vi "subHamamatsu_ApplyDAQwaveform.vi"(5 "Camera info":cluster{"Handle in":u32, "Image file path":path}, 6 "Acquisition params":T1={"Sampling rate (Hz)"=0.0, "dt (sec)"=0.0, "total time (sec)"=0.0, "# samples"=0, "Exposure time (ms)"=1000.0, "# frames"=0} {"Exposure time (ms)" format="%0.5f"; "Sampling rate (Hz)" format="%#.3f"}, 7 "Waveform port selection":T2={"Dev2 DO lines"=["Dev2/port0/line3", "Dev2/port0/line5"], "Dev2 AO lines"=["Dev2/ao3", "Dev2/ao5"], "Patch AO line"="Dev1/ao0", "Dev1 AI lines"=["Dev1/ai0", "Dev1/ai8"], "Dev1 timing DO"="Dev1/port0/line1", "Camera timing DI"="Dev1/port0/line0", "Dev1 trigger source"="/Dev1/PFI0", "Dev2 trigger source"="/Dev2/PFI0"}, 8 "Camera in (no error)":errorcluster, 9 "Dev1 AO waveform":waveform(dbl)(graph)={"t0"=timestamp(0 s since 1904-01-01), "dt"=0.1, "Y"=array[20000 elements]}, 10 "Dev2 AO waveform":waveform(dbl)[](graph)=[{"t0"=timestamp(0 s since 1904-01-01), "dt"=0.1, "Y"=array[20000 elements]}, {"t0"=timestamp(0 s since 1904-01-01), "dt"=0.1, "Y"=array[20000 elements]}], 11 "Dev2 DO waveform":digitalwaveform[](graph)=[{"t0"=timestamp(0 s since 1904-01-01), "dt"=0.1, "Y"={"transitions"=[0, 10000, 19999], "data"=[[1], [0], [0]]}}, {"t0"=timestamp(0 s since 1904-01-01), "dt"=0.1, "Y"={"transitions"=[0, 10000, 19999], "data"=[[0], [1], [1]]}}]) -> (0 "Camera out":errorcluster, 2 "AI Waveform":dbl[][](graph), 3 "Camera timging DI":digitalwaveform(graph))   [LabVIEW 2015]
uses:
  <vilib>/DAQmx/write.llb/DAQmx Write (Analog Wfm 1Chan NSamp).vi
  <vilib>/DAQmx/write.llb/DAQmx Write (Analog 1D Wfm NChan NSamp).vi
  <vilib>/DAQmx/write.llb/DAQmx Write (Digital 1D Wfm NChan NSamp).vi
  <vilib>/DAQmx/write.llb/DAQmx Write (Digital Wfm 1Chan NSamp).vi
  <vilib>/DAQmx/read.llb/DAQmx Read (Analog 2D DBL NChan NSamp).vi
  <vilib>/DAQmx/read.llb/DAQmx Read (Digital Wfm 1Chan NSamp).vi
  <vilib>/DAQmx/create/channels.llb/DAQmx Create Channel (DO-Digital Output).vi
  <vilib>/Waveform/DWDTOps.llb/DWDT Analog to Digital.vi
  <vilib>/DAQmx/create/channels.llb/DAQmx Create Channel (DI-Digital Input).vi
  <vilib>/DAQmx/create/channels.llb/DAQmx Create Channel (AO-Voltage-Basic).vi
  <vilib>/DAQmx/create/channels.llb/DAQmx Create Channel (AI-Voltage-Basic).vi
  <vilib>/DAQmx/configure/timing.llb/DAQmx Timing (Sample Clock).vi
  <vilib>/DAQmx/miscellaneous.llb/DAQmx Fill In Error Info.vi
  <vilib>/DAQmx/configure/trigger.llb/DAQmx Start Trigger (Digital Edge).vi
  <vilib>/Waveform/DWDTOps.llb/DWDT Uncompress Digital.vi
  <resource>/objmgr/daqmx.rc
panel:
  out "Dev1 SampClk.Rate":dbl format="%#.3f"
  out "Dev2 SampClk.Rate":dbl format="%#.3f"
  out "Dev1 timing DO":digitalwaveform(graph)={"t0"=timestamp(0 s since 1904-01-01), "dt"=0.1, "Y"={"transitions"=[0, 19999], "data"=[[1], [1]]}}
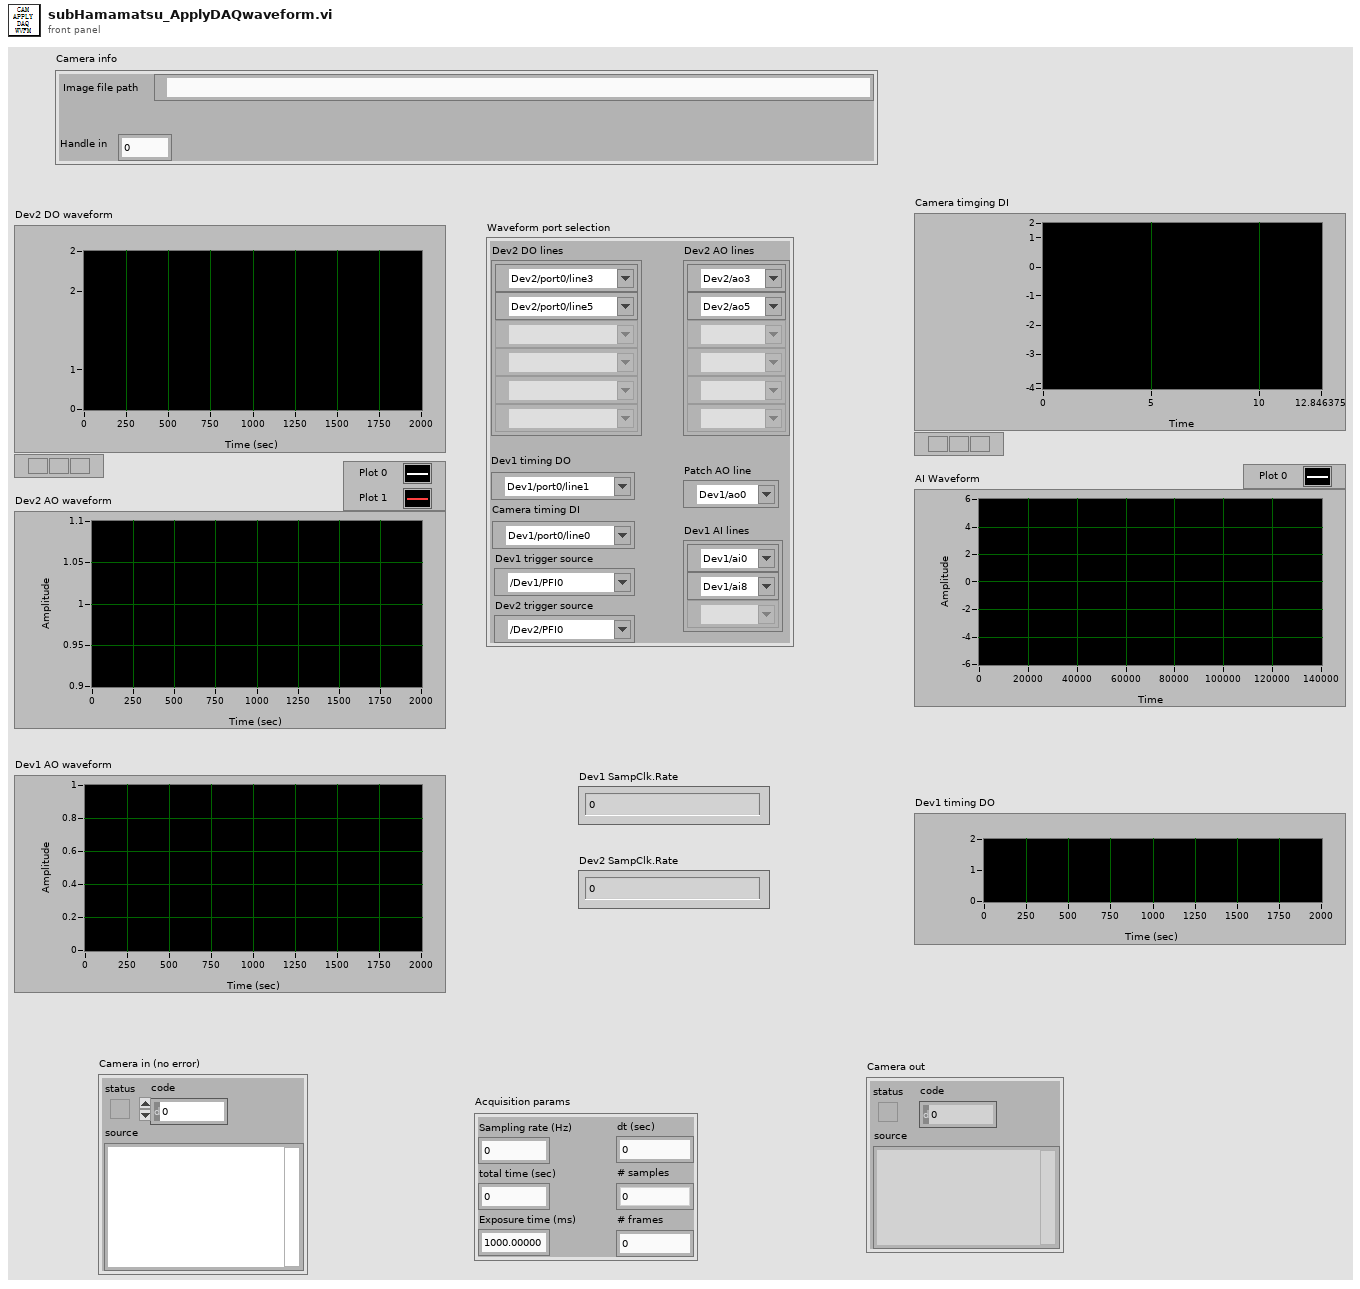
[diagram p1: front panel]
types:
  T1 = cluster{"Sampling rate (Hz)":dbl, "dt (sec)":dbl, "total time (sec)":dbl, "# samples":i32, "Exposure time (ms)":dbl, "# frames":i32}
  T2 = cluster{"Dev2 DO lines":tag[], "Dev2 AO lines":tag[], "Patch AO line":tag, "Dev1 AI lines":tag[], "Dev1 timing DO":tag, "Camera timing DI":tag, "Dev1 trigger source":tag, "Dev2 trigger source":tag}
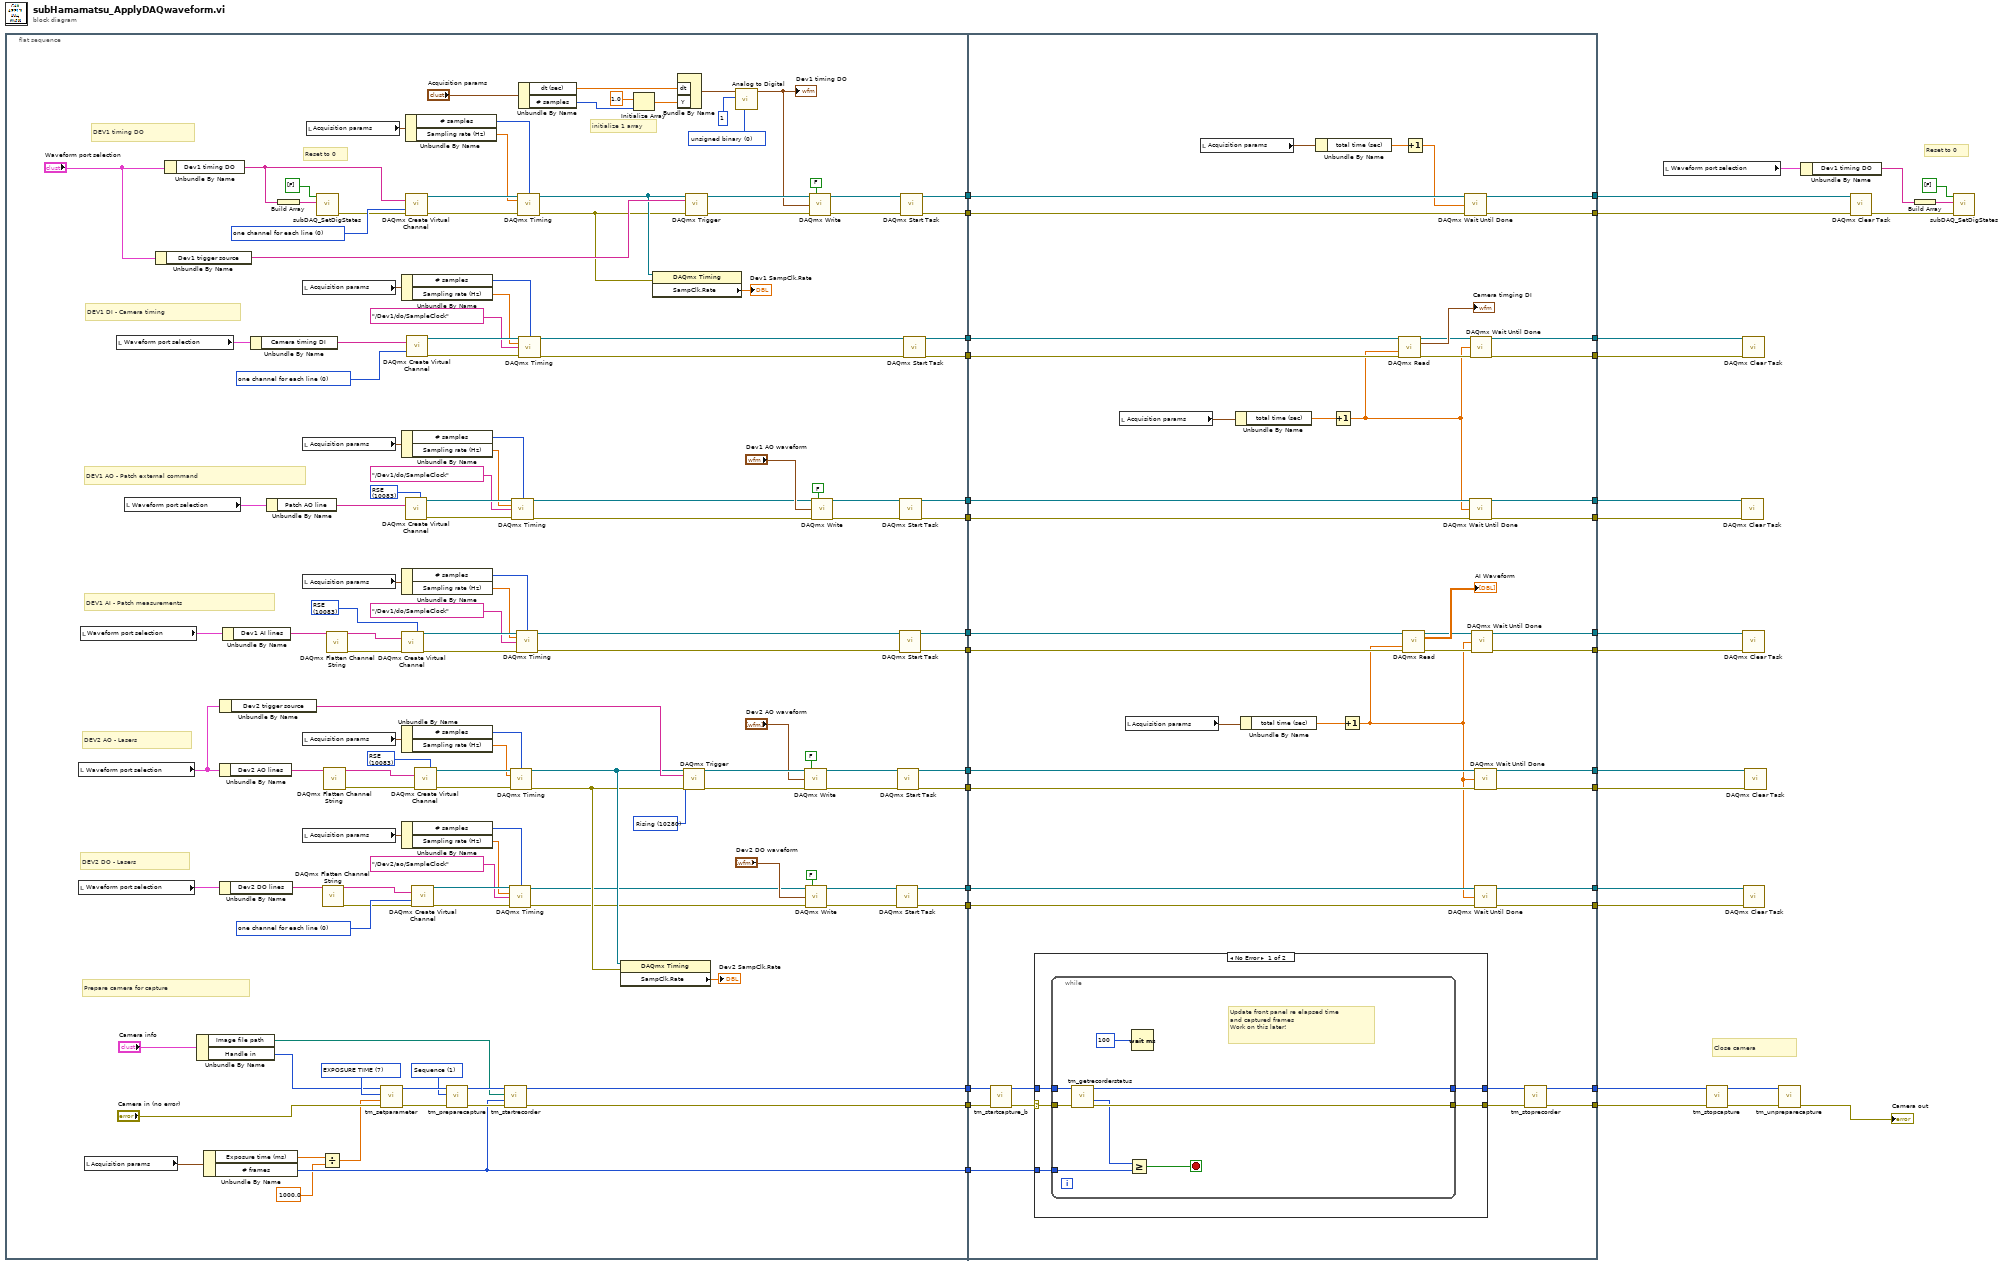
[diagram p0: block diagram]
diagram:
  # "Close camera"
  # "Reset to 0"
  n1 = flat-sequence {
    tunnel: [w155] -> w29
    tunnel: [w142] -> w28
    tunnel: [w141] -> w27
    tunnel: [w133] -> w26
    tunnel: [w122] -> w25
    tunnel: [w121] -> w24
    tunnel: [w114] -> w23
    tunnel: [w113] -> w22
    tunnel: [w110] -> w21
    tunnel: [w109] -> w20
    tunnel: [w106] -> w19
    tunnel: [w105] -> w18
    tunnel: [w91] -> w17
    tunnel: [w90] -> w16
    tunnel: [w65] -> w1
    tunnel: w29 -> [w204]
    tunnel: w28 -> [w206]
    tunnel: w27 -> [w205]
    tunnel: w26 -> [w203]
    tunnel: w25 -> [w202]
    tunnel: w24 -> [w201]
    tunnel: w23 -> [w199]
    tunnel: w22 -> [w200]
    tunnel: w21 -> [w198]
    tunnel: w20 -> [w197]
    tunnel: w19 -> [w196]
    tunnel: w18 -> [w195]
    tunnel: w17 -> [w216]
    tunnel: w16 -> [w215]
    tunnel: [w214] -> w15
    tunnel: [w213] -> w14
    tunnel: [w194] -> w13
    tunnel: [w193] -> w12
    tunnel: [w192] -> w11
    tunnel: [w191] -> w10
    tunnel: [w190] -> w9
    tunnel: [w189] -> w8
    tunnel: [w188] -> w7
    tunnel: [w187] -> w6
    tunnel: [w186] -> w5
    tunnel: [w185] -> w4
    tunnel: [w184] -> w3
    tunnel: [w183] -> w2
    tunnel: w1 -> [w182]
    frame #0 {
      w58 = 10083 items=["Default"=-1, "RSE"=10083, "Differential"=10106, "Pseudodifferential"=12529] ("output terminal configuration")
      w59 = 10083 items=["Default"=-1, "RSE"=10083, "Differential"=10106, "Pseudodifferential"=12529] ("output terminal configuration")
      w60 = 10083 items=["Default"=-1, "RSE"=10083, "NRSE"=10078, "Differential"=10106, "Pseudodifferential"=12529] ("input terminal configuration")
      w63 = 10280 items=["Rising"=10280, "Falling"=10171] ("edge")
      w89 = u16 0 items=["unsigned binary", "offset binary", "2's complement"] ("data format (offset binary)")
      w95 = 7 items=["BINNING"=1, "BITS PER CHANNEL"=2, "ACTIVE VIEW INDEX"=3, "CCD MODE"=4, "SENSOR MODE"=5, "READOUT MODE"=6, "EXPOSURE TIME"=7, "CONTRAST GAIN"=8, "CONTRAST OFFSET"=9, "LIGHT MODE"=10, "SENSITIVITY"=11, "WHITE BALANCE"=12, "PHOTON IMAGING MODE"=13, "HIGH DYNAMIC RANGE MODE"=14, "TRIGGER SOURCE"=15, "TRIGGER ACTIVE"=16, "TRIGGER MODE"=17, "TRIGGER POLARITY"=18, "TRIGGER GLOBAL EXPOSURE"=19, "FIRST TRIGGER BEHAVIOR"=20, "TRIGGER TIMES"=21, "OUTPUT TRIGGER POLARITY"=22, "OUTPUT TRIGGER DELAY"=23, "OUTPUT TRIGGER PERIOD"=24, "TEMPERATURE"=25, "TEMPERATURE TARGET"=26, "SENSOR COOLER FAN"=27, "MECHANICAL SHUTTER"=28, "BACK FOCUS POSITION"=29, "FRAMEBUNDLE MODE"=30, "FRAMEBUNDLE NUMBER"=31, "LINEBUNDLE HEIGHT"=32, "TRIGGER CONNECTOR"=33, "IMAGE PIXEL TYPE"=34] ("Parameter")
      w92 = 1 items=["Snap", "Sequence"] ("Capture mode")
      w146 = 0 items=["one channel for each line", "one channel for all lines"] ("line grouping")
      w159 = 0 items=["one channel for each line", "one channel for all lines"] ("line grouping")
      w172 = 0 items=["one channel for each line", "one channel for all lines"] ("line grouping")
      # "Prepare camera for capture"
      # "Reset to 0"
      # "DEV2 DO - Lasers"
      # "DEV2 AO - Lasers"
      # "DEV1 AI - Patch measurements"
      # "DEV1 AO - Patch external command"
      # "DEV1 DI - Camera timing"
      # "DEV1 timing DO"
      # "initialize 1 array"
      n2 = local read "Waveform port selection"() -> (w86:T2)
      n3 = local read "Waveform port selection"() -> (w108:T2)
      n4 = local read "Waveform port selection"() -> (w116:T2)
      n5 = local read "Acquisition params"() -> (w66:T1)
      n6 = local read "Waveform port selection"() -> (w135:T2)
      n7 = local read "Waveform port selection"() -> (w127:T2)
      n8 = Unbundle By Name("Waveform port selection") -> ("Dev1 trigger source"=w83:tag)
      n9 = Unbundle By Name("Waveform port selection") -> ("Dev1 timing DO"=w103:tag)
      n10 = Unbundle By Name("Camera info") -> ("Image file path"=w87:path, "Handle in"=w64:u32)
      n11 = Unbundle By Name(w66) -> ("Exposure time (ms)"=w39:dbl, "# frames"=w65:i32)
      n12 = Unbundle By Name(w86) -> ("Dev2 AO lines"=w111:tag[])
      n13 = Unbundle By Name(w108) -> ("Dev2 DO lines"=w107:tag[])
      n14 = Unbundle By Name(w86) -> ("Dev2 trigger source"=w85:tag)
      n15 = Unbundle By Name(w116) -> ("Dev1 AI lines"=w115:tag[])
      n16 = Unbundle By Name(w135) -> ("Camera timing DI"=w134:tag)
      n17 = Unbundle By Name(w127) -> ("Patch AO line"=w125:tag)
      n18 = Build Array(w103) -> (w102:tag[])
      n19 = local read "Acquisition params"() -> (w81:T1)
      n20 = local read "Acquisition params"() -> (w76:T1)
      n21 = local read "Acquisition params"() -> (w75:T1)
      n22 = local read "Acquisition params"() -> (w74:T1)
      n23 = local read "Acquisition params"() -> (w73:T1)
      n24 = local read "Acquisition params"() -> (w43:T1)
      n25 = call "subDAQ_SetDigStates.vi"("Digital line array"=w102, "Digital States (Value) array"=bool[] [FALSE] ("Digital state array")) -> ("Error out"=w104:errorcluster)  [unwired: 9 in]
      n26 = Divide(x=w39, y=1000.0) -> (x/y=w40:dbl)
      n27 = call <vilib>:"DAQmx Flatten Channel String.vi"("names in"=w107) -> ("names out"=w170:string, "error out"=w169:errorcluster)  [unwired: 13 in]
      n28 = call <vilib>:"DAQmx Flatten Channel String.vi"("names in"=w111) -> ("names out"=w151:string, "error out"=w152:errorcluster)  [unwired: 13 in]
      n29 = call <vilib>:"DAQmx Flatten Channel String.vi"("names in"=w115) -> ("names out"=w120:string, "error out"=w119:errorcluster)  [unwired: 13 in]
      n30 = call "tm_setparameter.vi"("error in (no error)"="Camera in (no error)", "Value in"=w40, "Parameter"=w95, "Handle in"=w64) -> ("error out"=w97:errorcluster, "Handle out"=w96:u32)  [unwired: 6 in]
      n31 = Unbundle By Name(w81) -> ("# samples"=w80:i32, "Sampling rate (Hz)"=w79:dbl)
      n32 = Unbundle By Name(w76) -> ("# samples"=w78:i32, "Sampling rate (Hz)"=w77:dbl)
      n33 = Unbundle By Name(w75) -> ("# samples"=w67:i32, "Sampling rate (Hz)"=w68:dbl)
      n34 = call-poly <vilib>:"DAQmx Create Virtual Channel.vi"("input terminal configuration"=w60, "physical channels"=w120, "error in"=w119) -> ("task out"=w117:refnum<k21>, "error out"=w118:errorcluster)  [unwired: 11 in]
      n35 = Unbundle By Name(w74) -> ("# samples"=w69:i32, "Sampling rate (Hz)"=w70:dbl)
      n36 = Unbundle By Name(w73) -> ("# samples"=w72:i32, "Sampling rate (Hz)"=w71:dbl)
      n37 = Unbundle By Name(w43) -> ("# samples"=w42:i32, "Sampling rate (Hz)"=w41:dbl)
      n38 = call-poly <vilib>:"DAQmx Create Virtual Channel.vi"("output terminal configuration"=w59, "physical channels"=w125) -> ("task out"=w128:refnum<k21>, "error out"=w130:errorcluster)  [unwired: 12 in]
      n39 = call-poly <vilib>:"DAQmx Create Virtual Channel.vi"("lines"=w103, "line grouping"=w146, "error in"=w104) -> ("task out"=w147:refnum<k21>, "error out"=w150:errorcluster)  [unwired: 11 in]
      n40 = call-poly <vilib>:"DAQmx Create Virtual Channel.vi"("lines"=w134, "line grouping"=w159) -> ("task out"=w158:refnum<k21>, "error out"=w157:errorcluster)  [unwired: 12 in]
      n41 = call-poly <vilib>:"DAQmx Create Virtual Channel.vi"("lines"=w170, "line grouping"=w172, "error in"=w169) -> ("task out"=w171:refnum<k21>, "error out"=w166:errorcluster)  [unwired: 11 in]
      n42 = call-poly <vilib>:"DAQmx Create Virtual Channel.vi"("output terminal configuration"=w58, "physical channels"=w151, "error in"=w152) -> ("task out"=w165:refnum<k21>, "error out"=w161:errorcluster)  [unwired: 11 in]
      n43 = call "tm_preparecapture.vi"("error in (no error)"=w97, "Capture mode"=w92, "Handle in"=w96) -> ("error out"=w93:errorcluster, "Handle out"=w94:u32)  [unwired: 5 in, 2 out]
      n44 = call "tm_startrecorder.vi"("error in (no error)"=w93, "frames"=w65, "File"=w87, "Handle in"=w94) -> ("error out"=w90:errorcluster, "Handle out"=w91:u32)  [unwired: 6 in]
      n45 = call-poly <vilib>:"DAQmx Timing.vi"("task/channels in"=w171, "samples per channel"=w72, "rate"=w71, "source"=tag "/Dev2/ao/SampleClock", "error in"=w166) -> ("task out"=w45:refnum<k21>, "error out"=w44:errorcluster)  [unwired: 9 in]
      n46 = call-poly <vilib>:"DAQmx Timing.vi"("task/channels in"=w165, "samples per channel"=w69, "rate"=w70, "error in"=w161) -> ("task out"=w52:refnum<k21>, "error out"=w51:errorcluster)  [unwired: 10 in]
      n47 = call-poly <vilib>:"DAQmx Timing.vi"("task/channels in"=w128, "samples per channel"=w78, "rate"=w77, "source"=tag "/Dev1/do/SampleClock", "error in"=w130) -> ("task out"=w55:refnum<k21>, "error out"=w54:errorcluster)  [unwired: 9 in]
      n48 = call-poly <vilib>:"DAQmx Timing.vi"("task/channels in"=w117, "samples per channel"=w67, "rate"=w68, "source"=tag "/Dev1/do/SampleClock", "error in"=w118) -> ("task out"=w47:refnum<k21>, "error out"=w46:errorcluster)  [unwired: 9 in]
      n49 = call-poly <vilib>:"DAQmx Timing.vi"("task/channels in"=w147, "samples per channel"=w42, "rate"=w41, "error in"=w150) -> ("task out"=w49:refnum<k21>, "error out"=w48:errorcluster)  [unwired: 10 in]
      n50 = Unbundle By Name("Acquisition params") -> ("dt (sec)"=w61:dbl, "# samples"=w62:i32)
      n51 = call-poly <vilib>:"DAQmx Timing.vi"("task/channels in"=w158, "samples per channel"=w80, "rate"=w79, "source"=tag "/Dev1/do/SampleClock", "error in"=w157) -> ("task out"=w57:refnum<k21>, "error out"=w56:errorcluster)  [unwired: 9 in]
      n52 = property class="DAQmx Timing"(reference=w52, error in=w51) -> ("SampClk.Rate"=→"Dev2 SampClk.Rate":dbl)  [unwired: 2 out]
      n53 = Initialize Array(1.0 ("element"), w62) -> (w139:dbl[])
      n54 = property class="DAQmx Timing"(reference=w49, error in=w48) -> ("SampClk.Rate"=→"Dev1 SampClk.Rate":dbl)  [unwired: 2 out]
      n55 = Bundle By Name("dt"=w61, "Y"=w139) -> (w137:waveform(dbl))  [unwired: 1 in]
      n56 = call-poly <vilib>:"DAQmx Trigger.vi"("task/channels in"=w52, "source"=w85, "edge"=w63, "error in"=w51) -> ("task out"=w163:refnum<k21>, "error out"=w162:errorcluster)  [unwired: 10 in]
      n57 = call-poly <vilib>:"DAQmx Trigger.vi"("task/channels in"=w49, "source"=w83, "error in"=w48) -> ("task out"=w144:refnum<k21>, "error out"=w145:errorcluster)  [unwired: 11 in]
      n58 = call-poly <vilib>:"Analog to Digital.vi"("data format (offset binary)"=w89, "resolution (16 bit)"=1, "analog waveform"=w137) -> ("digital waveform"=w136:digitalwaveform)  [unwired: 5 in, 3 out]
      "Dev1 timing DO" <- w136
      n59 = call-poly <vilib>:"DAQmx Write.vi"("task/channels in"=w163, "auto start"=FALSE, "data"="Dev2 AO waveform", "error in"=w162) -> ("task out"=w164:refnum<k21>, "error out"=w112:errorcluster)  [unwired: 9 in, 1 out]
      n60 = call-poly <vilib>:"DAQmx Write.vi"("task/channels in"=w45, "auto start"=FALSE, "data"="Dev2 DO waveform", "error in"=w44) -> ("task out"=w168:refnum<k21>, "error out"=w132:errorcluster)  [unwired: 9 in, 1 out]
      n61 = call-poly <vilib>:"DAQmx Write.vi"("task/channels in"=w144, "auto start"=FALSE, "data"=w136, "error in"=w145) -> ("task out"=w148:refnum<k21>, "error out"=w143:errorcluster)  [unwired: 9 in, 1 out]
      n62 = call-poly <vilib>:"DAQmx Write.vi"("task/channels in"=w55, "auto start"=FALSE, "data"="Dev1 AO waveform", "error in"=w54) -> ("task out"=w129:refnum<k21>, "error out"=w123:errorcluster)  [unwired: 9 in, 1 out]
      n63 = call <vilib>:"DAQmx Start Task.vi"("task/channels in"=w168, "error in"=w132) -> ("task out"=w106:refnum<k21>, "error out"=w105:errorcluster)  [unwired: 12 in]
      n64 = call <vilib>:"DAQmx Start Task.vi"("task/channels in"=w164, "error in"=w112) -> ("task out"=w110:refnum<k21>, "error out"=w109:errorcluster)  [unwired: 12 in]
      n65 = call <vilib>:"DAQmx Start Task.vi"("task/channels in"=w47, "error in"=w46) -> ("task out"=w113:refnum<k21>, "error out"=w114:errorcluster)  [unwired: 12 in]
      n66 = call <vilib>:"DAQmx Start Task.vi"("task/channels in"=w129, "error in"=w123) -> ("task out"=w122:refnum<k21>, "error out"=w121:errorcluster)  [unwired: 12 in]
      n67 = call <vilib>:"DAQmx Start Task.vi"("task/channels in"=w148, "error in"=w143) -> ("task out"=w142:refnum<k21>, "error out"=w141:errorcluster)  [unwired: 12 in]
      n68 = call <vilib>:"DAQmx Start Task.vi"("task/channels in"=w57, "error in"=w56) -> ("task out"=w155:refnum<k21>, "error out"=w133:errorcluster)  [unwired: 12 in]
    }
    frame #1 {
      n69 = call "tm_startcapture_b.vi"("error in (no error)"=w215, "Handle in"=w216) -> ("error out"=w217:errorcluster, "Handle out"=w218:u32)  [unwired: 8 in]
      n70 = case shown="No Error" w217 {
        selector: w217 -> [w225 w234]
        tunnel: w218 -> [w224 w235]
        tunnel: [w222 w235] -> w220
        tunnel: [w223 w234] -> w219
        tunnel: w182 -> [w221 _]
        frame No Error {
          n71 = while {
            tunnel: w225 -> [w232]
            tunnel: w224 -> [w231]
            tunnel: [w230] -> w223
            tunnel: [w233] -> w222
            tunnel: w221 -> [w226]
            stop <- w229 stop-if-true
            # "Update front panel re elapsed time\nand captured frames\nWork on this later!"
            n72 = call "tm_getrecorderstatus.vi"("error in (no error)"=w232, "Handle"=w231) -> ("error out"=w230:errorcluster, "Count"=w227:i32, "Handle"=w233:u32)  [unwired: 6 in, 1 out]
            n73 = Greater Or Equal?(x=w227, y=w226) -> (x >= y?=w229:bool)
            n74 = Wait (ms)(milliseconds to wait=u32 100) -> ()  [unwired: 1 out]
          }
        }
        frame Error {
        }
      }
      n75 = local read "Acquisition params"() -> (w176:T1)
      n76 = local read "Acquisition params"() -> (w174:T1)
      n77 = local read "Acquisition params"() -> (w178:T1)
      n78 = Unbundle By Name(w176) -> ("total time (sec)"=w175:dbl)
      n79 = Unbundle By Name(w174) -> ("total time (sec)"=w173:dbl)
      n80 = Unbundle By Name(w178) -> ("total time (sec)"=w177:dbl)
      n81 = Increment(x=w175) -> (x+1=w180:dbl)
      n82 = Increment(x=w173) -> (x+1=w179:dbl)
      n83 = call-poly <vilib>:"DAQmx Read.vi"("task/channels in"=w204, "timeout"=w180, "error in"=w203) -> ("task out"=w209:refnum<k21>, "data"=→"Camera timging DI":digitalwaveform, "error out"=w212:errorcluster)  [unwired: 10 in]
      n84 = call-poly <vilib>:"DAQmx Read.vi"("task/channels in"=w200, "timeout"=w179, "error in"=w199) -> ("task out"=w207:refnum<k21>, "data"=→"AI Waveform":dbl[][], "error out"=w208:errorcluster)  [unwired: 10 in]
      n85 = Increment(x=w177) -> (x+1=w181:dbl)
      n86 = call <vilib>:"DAQmx Wait Until Done.vi"("task/channels in"=w206, "timeout (sec)"=w181, "error in"=w205) -> ("task out"=w194:refnum<k21>, "error out"=w193:errorcluster)  [unwired: 11 in]
      n87 = call <vilib>:"DAQmx Wait Until Done.vi"("task/channels in"=w202, "timeout (sec)"=w180, "error in"=w201) -> ("task out"=w190:refnum<k21>, "error out"=w189:errorcluster)  [unwired: 11 in]
      n88 = call <vilib>:"DAQmx Wait Until Done.vi"("task/channels in"=w209, "timeout (sec)"=w180, "error in"=w212) -> ("task out"=w192:refnum<k21>, "error out"=w191:errorcluster)  [unwired: 11 in]
      n89 = call <vilib>:"DAQmx Wait Until Done.vi"("task/channels in"=w207, "timeout (sec)"=w179, "error in"=w208) -> ("task out"=w188:refnum<k21>, "error out"=w187:errorcluster)  [unwired: 11 in]
      n90 = call <vilib>:"DAQmx Wait Until Done.vi"("task/channels in"=w198, "timeout (sec)"=w179, "error in"=w197) -> ("task out"=w186:refnum<k21>, "error out"=w185:errorcluster)  [unwired: 11 in]
      n91 = call <vilib>:"DAQmx Wait Until Done.vi"("task/channels in"=w196, "timeout (sec)"=w179, "error in"=w195) -> ("task out"=w184:refnum<k21>, "error out"=w183:errorcluster)  [unwired: 11 in]
      n92 = call "tm_stoprecorder.vi"("error in (no error)"=w219, "Handle in"=w220) -> ("error out"=w213:errorcluster, "Handle out"=w214:u32)  [unwired: 8 in]
    }
  }
  n93 = local read "Waveform port selection"() -> (w35:T2)
  n94 = call "tm_stopcapture.vi"("error in (no error)"=w14, "Handle in"=w15) -> ("error out"=w32:errorcluster, "Handle out"=w31:u32)  [unwired: 8 in]
  n95 = call <vilib>:"DAQmx Clear Task.vi"("task in"=w9, "error in"=w8) -> ()  [unwired: 13 in, 1 out]
  n96 = call <vilib>:"DAQmx Clear Task.vi"("task in"=w11, "error in"=w10) -> ()  [unwired: 13 in, 1 out]
  n97 = call <vilib>:"DAQmx Clear Task.vi"("task in"=w7, "error in"=w6) -> ()  [unwired: 13 in, 1 out]
  n98 = call <vilib>:"DAQmx Clear Task.vi"("task in"=w3, "error in"=w2) -> ()  [unwired: 13 in, 1 out]
  n99 = call <vilib>:"DAQmx Clear Task.vi"("task in"=w5, "error in"=w4) -> ()  [unwired: 13 in, 1 out]
  n100 = call "tm_unpreparecapture.vi"("error in (no error)"=w32, "Handle in"=w31) -> ("error out"=→"Camera out":errorcluster)  [unwired: 8 in, 1 out]
  n101 = Unbundle By Name(w35) -> ("Dev1 timing DO"=w33:tag)
  n102 = call <vilib>:"DAQmx Clear Task.vi"("task in"=w13, "error in"=w12) -> ("error out"=w34:errorcluster)  [unwired: 13 in]
  n103 = Build Array(w33) -> (w36:tag[])
  n104 = call "subDAQ_SetDigStates.vi"("Error in (no error)"=w34, "Digital line array"=w36, "Digital States (Value) array"=bool[] [FALSE] ("Digital state array")) -> ()  [unwired: 8 in, 1 out]
